vi "ScaleForce.vi"(6 "Scale Dir":T1=enum."Full scale -> Model scale", 8 "Scale factor":dbl, 11 "Force (In)":dbl) -> (3 "Force (Out)":dbl)   [LabVIEW 2018]
uses:
  Clusters/ScalingEnum.ctl
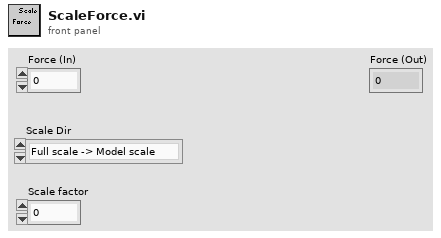
[diagram p1: front panel]
types:
  T1 = typedef "ScalingEnum.ctl" = enum16{"Model scale -> Full scale", "Full scale -> Model scale"}
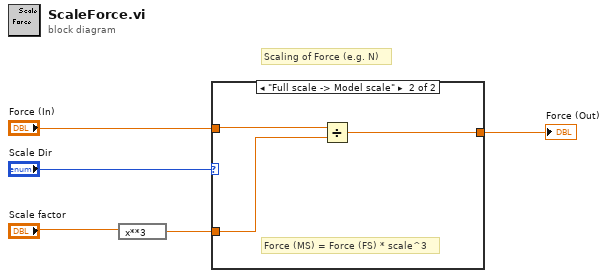
[diagram p0: block diagram]
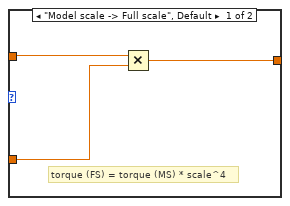
[diagram p2: hidden frame]
diagram:
  # "Scaling of Force (e.g. N)"
  n1 = expression code="x**3"("Scale factor") -> (w2:dbl)
  n2 = case shown="\"Full scale -> Model scale\"" "Scale Dir" {
    tunnel: "Force (In)" -> [w8 w11]
    tunnel: w2 -> [w7 w10]
    tunnel: [w6 w9] -> w3
    frame "Model scale -> Full scale", Default {
      # "torque (FS) = torque (MS) * scale^4"
      n3 = Multiply(x=w8, y=w7) -> (x*y=w6:dbl)
    }
    frame "Full scale -> Model scale" {
      # "Force (MS) = Force (FS) * scale^3"
      n4 = Divide(x=w11, y=w10) -> (x/y=w9:dbl)
    }
  }
  "Force (Out)" <- w3
